vi "Timer Reached Next State With Stop.vi"(6 "Stop":bool, 7 "Time has Elapsed":bool, 9 "Stop State":T1, 10 "Next State":T1=enum."#3 Run", 11 "Status Out输入":T2={"State"=enum."Idle", "Motor"={"#1"=FALSE, "#2"=FALSE, "#3"=FALSE}, "Timer"=30.0}) -> (3 "Status Out输出":T2={"State"=enum."Idle", "Motor"={"#1"=FALSE, "#2"=FALSE, "#3"=FALSE}, "Timer"=30.0})   [LabVIEW 2013]
uses:
  Control/Data.ctl
  Control/State.ctl
  Control/Motor.ctl
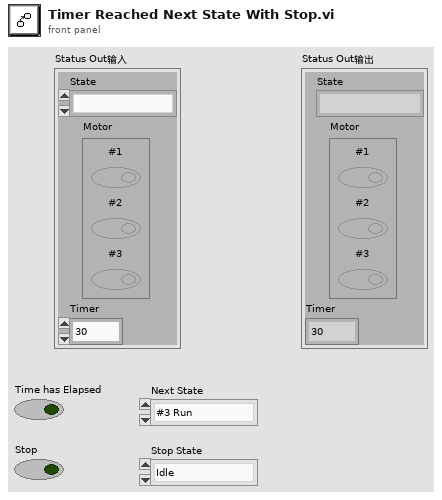
[diagram p1: front panel]
types:
  T1 = typedef "State.ctl" = enum16{"Idle", "#1 Run", "#2 Run", "#3 Run", "#3 Stop", "#2 Stop", "#1 Stop"}
  T2 = typedef "Data.ctl" = cluster{"State":T1, "Motor":T3, "Timer":dbl}
  T3 = typedef "Motor.ctl" = cluster{"#1":bool, "#2":bool, "#3":bool}
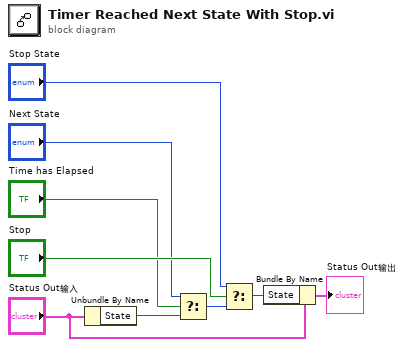
[diagram p0: block diagram]
diagram:
  n1 = Unbundle By Name("Status Out输入") -> ("State"=w4:T1)
  n2 = Select(t="Next State", s="Time has Elapsed", f=w4) -> (s? t:f=w9:T1)
  n3 = Select(t="Stop State", s="Stop", f=w9) -> (s? t:f=w7:T1)
  n4 = Bundle By Name(cluster="Status Out输入", "State"=w7) -> (→"Status Out输出":T2)
